vi "Get Limits.vi"(8 "error in (no error)":errorcluster, 10 "Axis":T1 items=["1"=1, "2"=2, "3"=3, "4"=4], 11 "DelayLine in":refnum<class "DelayLine.lvclass">) -> (0 "error out":errorcluster, 1 "max":dbl, 2 "min":dbl, 3 "DelayLine out":refnum<class "DelayLine.lvclass">, 4 "real pos":dbl)   [LabVIEW 2015]
uses:
  DelayLine.lvclass
  DelayLineLS4/LS4 axis.ctl
  DelayLineLS4/LS4_parameters.ctl
  GeneralFunctionality/GeneralFunctionality.lvclass/GeneralFunctionality.ctl
  Config/Config.lvclass
  GeneralFunctionality/GeneralFunctionality.lvclass
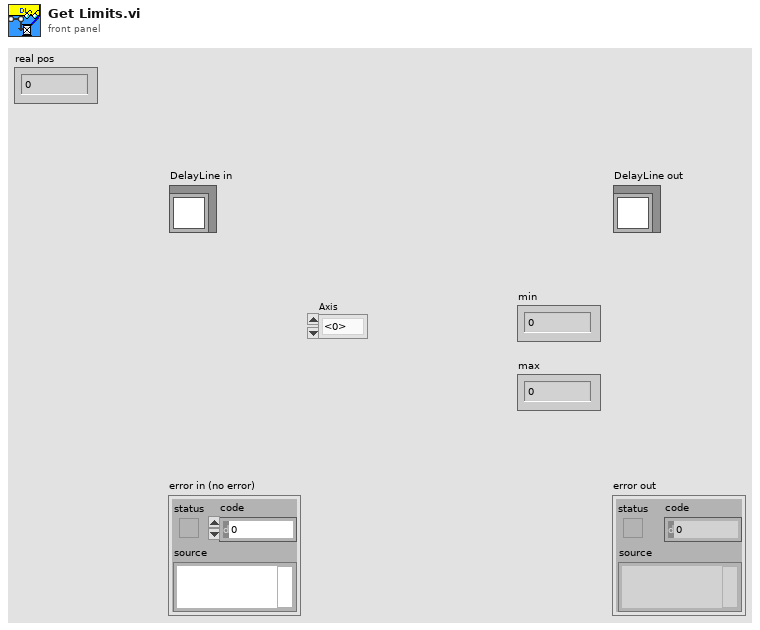
[diagram p1: front panel]
types:
  T1 = typedef "DelayLine.lvclass/LS4 axis.ctl" = u16
  T2 = typedef "DelayLine.lvclass/LS4_parameters.ctl" = string
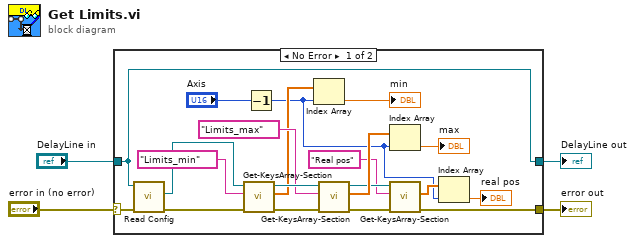
[diagram p0: block diagram]
diagram:
  n1 = case shown="No Error" "error in (no error)" {
    selector: "error in (no error)" -> [w13 w26]
    tunnel: [w9 w26] -> w3
    tunnel: [w12 w25] -> w1
    tunnel: "DelayLine in" -> [w12 w25]
    frame No Error {
      n2 = call "Read Config.vi"("error in (no error)"=w13, "GeneralFunctionality en entrée"=w12) -> ("error out"=w23:errorcluster, "Config.lvclass"=w24:refnum<class "Config.lvclass">)  [unwired: 7 in, 1 out]
      n3 = call "Get-KeysArray-Section.vi"("error in (no error)"=w23, "Section"=T2 "Limits_min", "Config in"=w24) -> ("error out"=w20:errorcluster, "Array"=w17:dbl[], "Config out"=w21:refnum<class "Config.lvclass">)  [unwired: 6 in]
      n4 = Decrement(x="Axis") -> (x-1=w5:T1)
      n5 = Index Array(array=w17, index=w5) -> (element=→"min":dbl)
      n6 = call "Get-KeysArray-Section.vi"("error in (no error)"=w20, "Section"=T2 "Limits_max", "Config in"=w21) -> ("error out"=w6:errorcluster, "Array"=w18:dbl[], "Config out"=w10:refnum<class "Config.lvclass">)  [unwired: 6 in]
      n7 = Index Array(array=w18, index=w5) -> (element=→"max":dbl)
      n8 = call "Get-KeysArray-Section.vi"("error in (no error)"=w6, "Section"="Real pos", "Config in"=w10) -> ("error out"=w9:errorcluster, "Array"=w8:dbl[])  [unwired: 6 in, 1 out]
      n9 = Index Array(array=w8, index=w5) -> (element=→"real pos":dbl)
    }
    frame Error {
    }
  }
  "error out" <- w3
  "DelayLine out" <- w1
